vi "Diff to Right Arm Motor.vi"(9 "Right Pot":dbl, 10 "Left Pot":dbl, 11 "Joystick Axis":dbl) -> (3 "Right Arm Motor Axis":dbl)   [LabVIEW 2014]
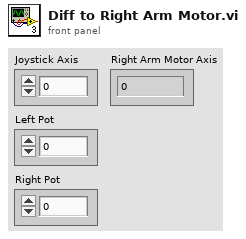
[diagram p1: front panel]
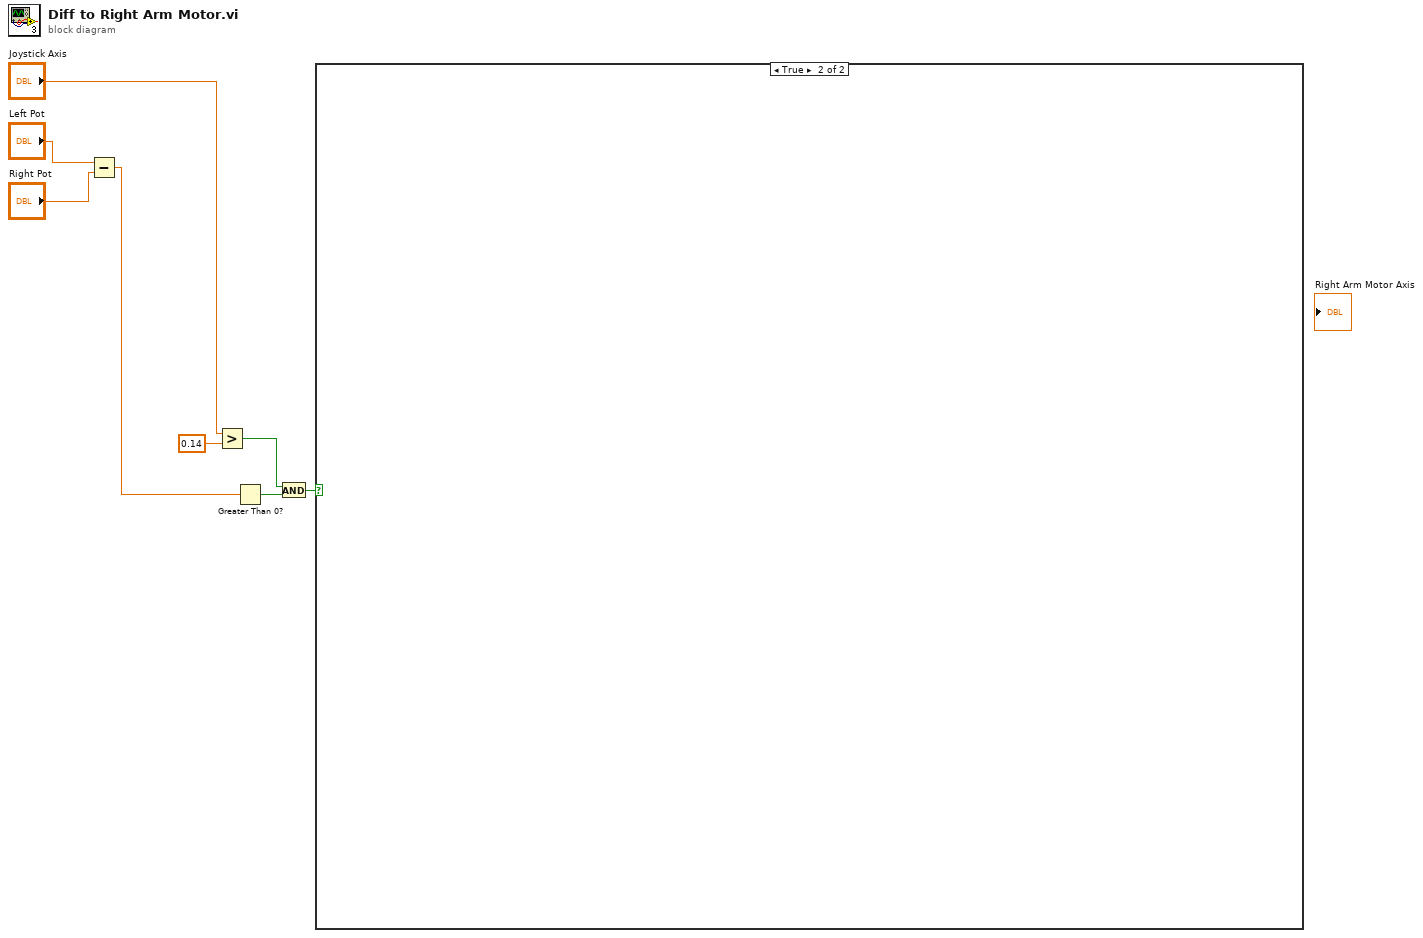
[diagram p0: block diagram]
diagram:
  n1 = Subtract(x="Left Pot", y="Right Pot") -> (x-y=w1:dbl)
  n2 = Greater?(x="Joystick Axis", y=0.14) -> (0:w3:bool)
  n3 = Greater Than 0?(x=w1) -> (x > 0?=w2:bool)
  n4 = And(x=w3, y=w2) -> (x .and. y?=w4:bool)
  n5 = case shown="True" w4 {
    frame False {
      n6 = case shown="False" {
        selector: _ -> [_ _]
        frame False {
          n7 = case shown="False" {
            selector: _ -> [_ _]
            frame False {
              n8 = case shown="False" {
                selector: _ -> [_ _]
                frame False {
                  n9 = case shown="False" {
                    selector: _ -> [_ _]
                    frame False {
                      n10 = case shown="False" {
                        selector: _ -> [_ _]
                        frame False {
                          n11 = case shown="True" {
                            selector: _ -> [_ _]
                            frame False {
                            }
                            frame True {
                            }
                          }
                        }
                        frame True {
                        }
                      }
                    }
                    frame True {
                    }
                  }
                }
                frame True {
                }
              }
            }
            frame True {
            }
          }
        }
        frame True {
        }
      }
    }
    frame True {
    }
  }
